vi "Conductus Read Set Point.vi"(1 "VISA session":refnum<visa-resource-name>) -> (0 "?":dbl format="%.2e")   [LabVIEW 2019]
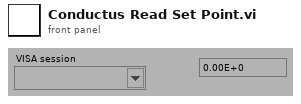
[diagram p1: front panel]
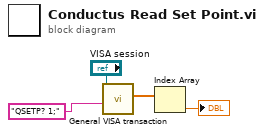
[diagram p0: block diagram]
diagram:
  n1 = call "General VISA transaction.vi"("Command String"="QSETP? 1;", "VISA Session"="VISA session") -> ("Measurement"=w2:dbl[])  [unwired: 4 in, 5 out]
  n2 = Index Array(array=w2) -> (element=→"?":dbl)  [unwired: 1 in]
